vi "Inspect.vi"(10 "Msg Strategy in":refnum<class "Msg Strategy.lvclass">, 11 "Base jettl in":refnum<class "Base jettl.lvclass">) -> (2 "Msg Strategy out":refnum<class "Msg Strategy.lvclass">, 3 "Base jettl out":refnum<class "Base jettl.lvclass">)   [LabVIEW 2021, in "jettl.lvlib" / "Base jettl.lvclass"]
uses:
  Base jettl.lvclass
  Msg Strategy/Msg Strategy.lvclass
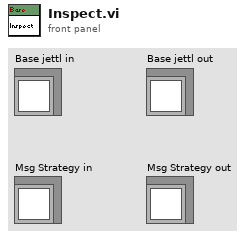
[diagram p1: front panel]
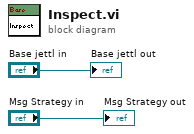
[diagram p0: block diagram]
diagram:
  "Base jettl out" <- "Base jettl in"
  "Msg Strategy out" <- "Msg Strategy in"
